vi "Create Python TCP Server.vi"(7 "net address (0: Listen on All Adaptors)":u32, 8 "error in (no error)":errorcluster, 9 "max connections (0: no limit)":u32, 10 "TCP port":u16) -> (0 "error out":errorcluster, 2 "Python Method Call":refnum<user-event>, 3 "TCP Server RefNum":T1)   [LabVIEW 2013, in "JKI_Python_Bridge_for_LV.lvlib" / "Server.lvclass"]
uses:
  Server.lvclass
  Call/Call.lvclass
  <vilib>/addons/_JKI.lib/_jki_lib_tcp_server.llb/TCP Server Object RefNum__jki_lib_tcp_server.ctl
  <vilib>/addons/_JKI.lib/_jki_lib_tcp_server.llb/TCP Server Object RefNum - Enum__jki_lib_tcp_server.ctl
panel:
  # "Copyright © 2004-2008 JKI. All rights reserved.\n\nAuthor: Jim Kring [jim.kring@jameskring.com]\n\nThis library is provided \"AS IS\" ,WITHOUT WARRANTIES OR \nCONDITIONS OF ANY KIND, either express or implied.\n\nJames Kring, Inc. -- http://www.jameskring.com"
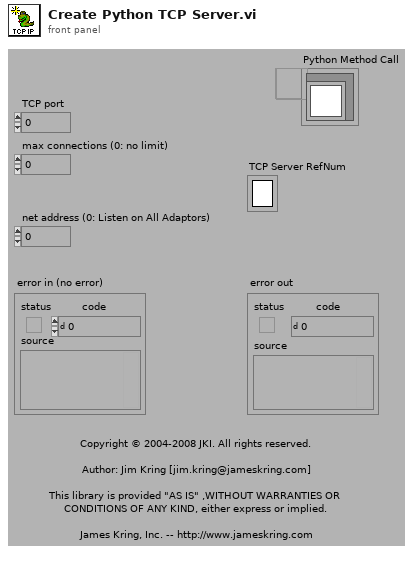
[diagram p1: front panel]
types:
  T1 = typedef "TCP Server Object RefNum__jki_lib_tcp_server.ctl" = refnum<k1>
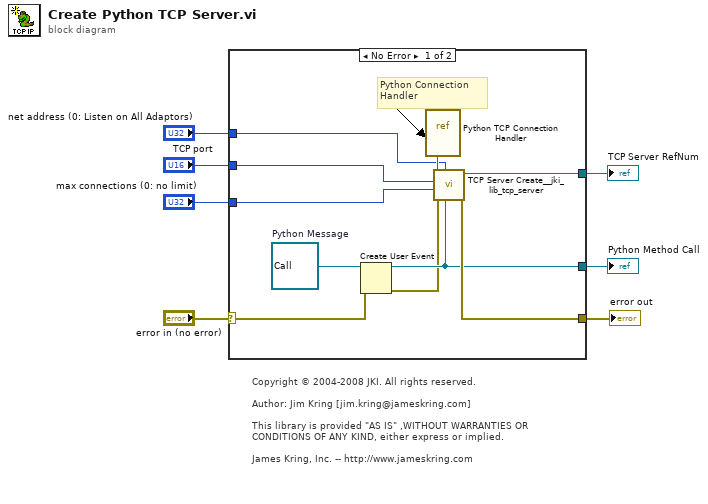
[diagram p0: block diagram]
diagram:
  # "Copyright © 2004-2008 JKI. All rights reserved.\n\nAuthor: Jim Kring [jim.kring@jameskring.com]\n\nThis library is provided \"AS IS\" ,WITHOUT WARRANTIES OR \nCONDITIONS OF ANY KIND, either express or implied.\n\nJames Kring, Inc. -- http://www.jameskring.com"
  n1 = case shown="No Error" "error in (no error)" {
    selector: "error in (no error)" -> [w12 w18]
    tunnel: [w16 w18] -> w4
    tunnel: [w15 _] -> w5
    tunnel: [w14 _] -> w6
    tunnel: "max connections (0: no limit)" -> [w11 _]
    tunnel: "TCP port" -> [w10 _]
    tunnel: "net address (0: Listen on All Adaptors)" -> [w9 _]
    frame No Error {
      w8 = refnum<class "Call.lvclass"> refnum  # Python Message
      # "Python Connection \nHandler"
      n2 = Create User Event(user event datatype=w8, error in=w12) -> (user event=w14:refnum<user-event>, error out=w13:errorcluster)
      n3 = vi-ref "Python TCP Connection Handler.vi"() -> ("vi reference"=w17:refnum<vi>)
      n4 = call <vilib>:"TCP Server Create__jki_lib_tcp_server.vi"("Additional Data"=w14, "net address (0: Listen on All Adaptors)"=w9, "error in (no error)"=w13, "max connections (0: no limit)"=w11, "port"=w10, "Connection Handler Call-Back VI RefNum"=w17) -> ("error out"=w16:errorcluster, "TCP Server RefNum"=w15:T1)  [unwired: 4 out]
    }
    frame Error {
    }
  }
  "Python Method Call" <- w6
  "TCP Server RefNum" <- w5
  "error out" <- w4
